vi "AlazarStackChannels1Pass.vi"(6 "AlazarCluster":T8, 7 "Digitizer Settings":T4 {"Trigger Settings"."Trig Slope" items=["Positive", "Negative"]; "Trigger Settings"."Level (mV)" format="%.2f"; "Trigger Settings"."Trig Coupling" items=["DC 1 MOhm", "AC 1 MOhm", "DC 50 Ohm", "AC 50 Ohm"]; "Trigger Settings"."Trig Source" items=["Chan 1", "External"]; "Rel Dig Delay" format="%.2f"; "DigTimeOut" format="%.2f"; "Avg Num" min=1; "Offset delay (us)" format="%.2f"; "Additional dig delay (us)" format="%.2f"; "Digitizer delay (us)" format="%.2f"}, 8 "error in":errorcluster, 10 "Extra Shift":u16, 11 "Ann Array Params":T1={"Synth Foc?"=FALSE, "Focal Zones"=41, "Switch T/R"=0, "Trans Geometry (mm)"={"Transducer"=0, "Geo Focus"=12.0, "a (radius)"=3.0, "# of rings"=5, "kerf space "=0.1, "Center Freq"=12.0}, "Sub Ap Excite?"=FALSE, "Full Array Scan?"=FALSE, "Xmt/Rcv"={"XMIT"=[TRUE, TRUE, TRUE, TRUE, TRUE], "RCV"=[TRUE, TRUE, TRUE, TRUE, TRUE]}, "PulseSpacing (us)"=0.0, "Xmit Ring"=0, "XMIT CHS"=0, "RCV CHS"=0, "GPU?"=FALSE, "Save TIFF?"=FALSE, "downfactor"=1, "RCV 1CH"=0} {"RCV 1CH" items=["All", "1", "2", "3", "4", "5"]; "Trans Geometry (mm)"."Transducer" items=["6D 12R 40 MHz"=0, "10D 31R 20 MHz"=1, "10D 23R 20 MHz"=2, "6D 23R 40 MHz"=3, "4.5D 10.7R 40 MHz"=4, "9D 23.5R 20 MHz"=5, "9D 25.8R 20MHz"=6, "Enter"=99]; "Switch T/R" min=1 max=5 step=1}) -> (0 "error out":errorcluster, 1 "Voltage Scale":dbl, 2 "Return Code":u32, 3 "DataInterleavedOut":i16[](array[numeric]), 4 "DeInterleaved":i16[](array[numeric]))   [LabVIEW 2022 SP3]
uses:
  -DigitizerRoutines/DigitizerSettings.ctl
  -DigitizerRoutines/Digitizer.ctl
  -DigitizerRoutines/DigConfig.ctl
  -DigitizerRoutines/DigitizerID.ctl
  C:/Windows/System32/ADQAPI_dotNet_helper.dll
  Annular Array/-AnnularRoutines/AnnularArray.ctl
  Annular Array/-AnnularRoutines/TransGeometry.ctl
  Annular Array/-AnnularRoutines/ArrayGeometry.ctl
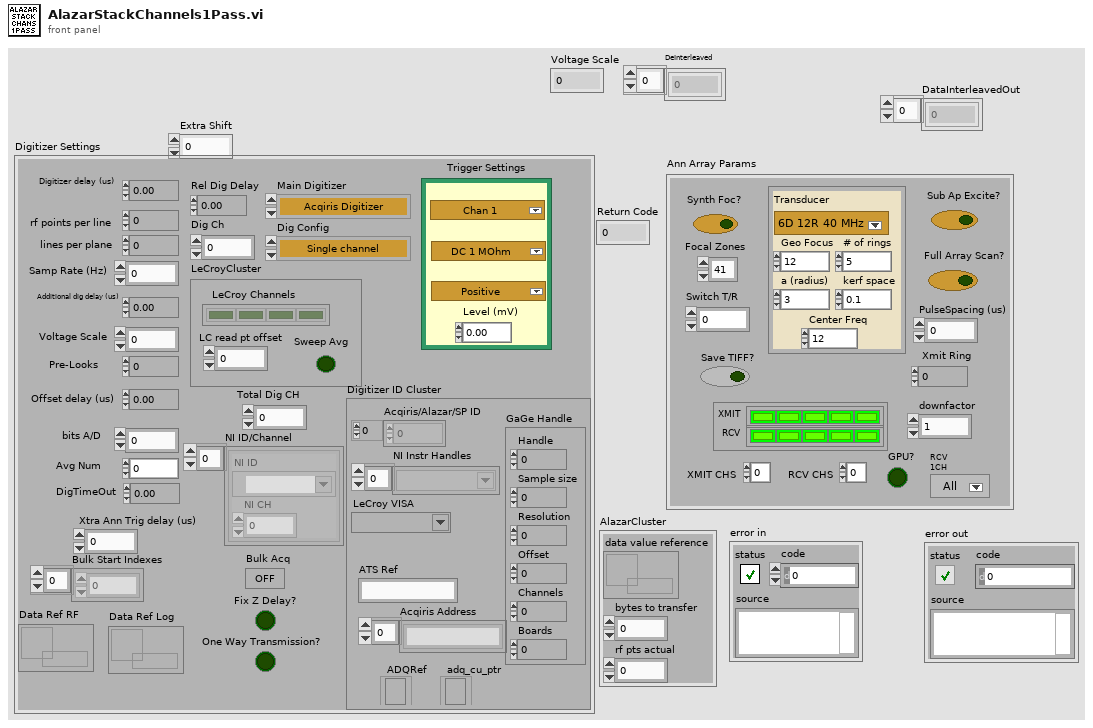
[diagram p1: front panel]
types:
  T1 = typedef "AnnularArray.ctl" = cluster{"Synth Foc?":bool, "Focal Zones":i16, "Switch T/R":i16, "Trans Geometry (mm)":T2, "Sub Ap Excite?":bool, "Full Array Scan?":bool, "Xmt/Rcv":cluster{"XMIT":bool[], "RCV":bool[]}, "PulseSpacing (us)":sgl, "Xmit Ring":i32, "XMIT CHS":u8, "RCV CHS":u8, "GPU?":bool, "Save TIFF?":bool, "downfactor":i32, "RCV 1CH":u16}
  T2 = typedef "TransGeometry.ctl" = cluster{"Transducer":T3, "Geo Focus":dbl, "a (radius)":dbl, "# of rings":i32, "kerf space ":dbl, "Center Freq":dbl}
  T3 = typedef "ArrayGeometry.ctl" = u16
  T4 = typedef "DigitizerSettings.ctl" = cluster{"Digitizer delay (us) ":dbl, "rf points per line":i32, "lines per plane":i32, "Samp Rate (Hz)":dbl, "Additional dig delay (us)":dbl, "Voltage Scale":dbl, "Pre-Looks":i32, "Offset delay (us)":dbl, "bits A/D":i8, "Avg Num":i32, "DigTimeOut":sgl, "Rel Dig Delay":sgl, "Dig Ch":i32, "LeCroyCluster":cluster{"LeCroy Channels":bool[], "LC read pt offset":dbl, "Sweep Avg":bool}, "Main Digitizer":T5, "Dig Config":T6, "Digitizer ID Cluster":T7, "Trigger Settings":cluster{"Trig Source":u16, "Trig Coupling":u16, "Trig Slope":u16, "Level (mV)":dbl}, "Bulk Acq":bool, "Bulk Start Indexes":i32[], "Data Ref RF":refnum<data-value>, "NI ID/Channel":cluster{"NI ID":refnum<k15>, "NI CH":i32}[], "Total Dig CH":i32, "Xtra Ann Trig delay (us)":dbl, "Fix Z Delay?":bool, "One Way Transmission?":bool, "Data Ref Log":refnum<data-value>}
  T5 = typedef "Digitizer.ctl" = enum16{"Acqiris Digitizer", "NI Digitizer", "LeCroy", "GaGe", "AlazarTech", "No Digitizer", "Teledyne"}
  T6 = typedef "DigConfig.ctl" = enum16{"Single channel", "2 Chans w/ 2 Acqiris", "2 Chans w/ 1 Acqiris", "5-CH Pulser New", "5-CH pulser w/ ann array", "5-pass style ann array", "Empty"}
  T7 = typedef "DigitizerID.ctl" = cluster{"Acqiris/Alazar/SP ID":u32[], "NI Instr Handles":refnum<k15>[], "LeCroy VISA":refnum<visa-resource-name>, "GaGe Handle":cluster{"Handle":u32, "Sample size":u32, "Resolution":i32, "Offset":i32, "Channels":u32, "Boards":u32}, "ATS Ref":string, "Acqiris Address":string[], "ADQRef":refnum<k24>, "adq_cu_ptr":refnum<k24>}
  T8 = cluster{"data value reference":refnum<data-value>, "bytes to transfer":u32, "rf pts actual":u32}
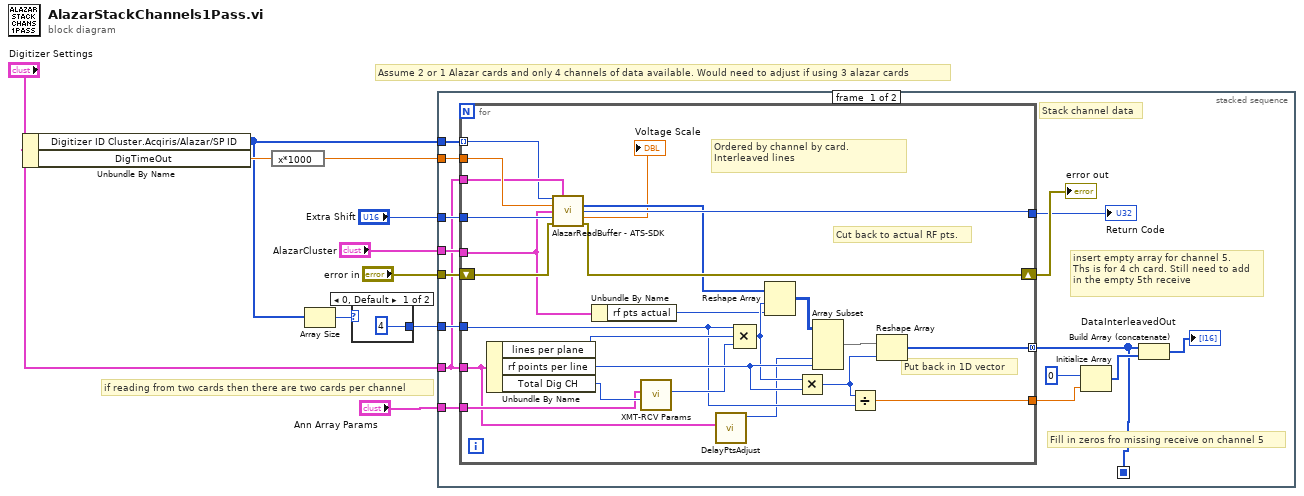
[diagram p0: block diagram]
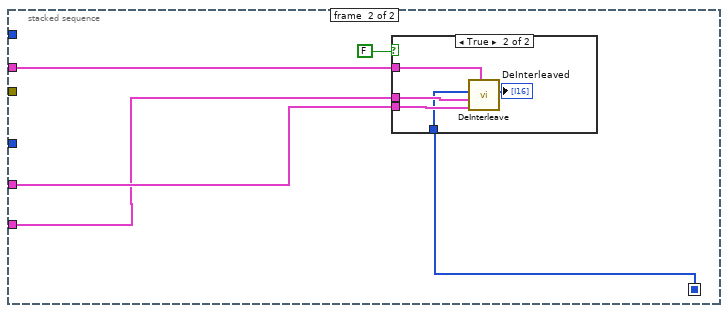
[diagram p2: hidden frame]
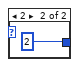
[diagram p4: hidden frame]
diagram:
  # "Assume 2 or 1 Alazar cards and only 4 channels of data available. Would need to adjust if using 3 alazar cards"
  # "if reading from two cards then there are two cards per channel"
  n1 = Unbundle By Name("Digitizer Settings") -> ("Digitizer ID Cluster.Acqiris/Alazar/SP ID"=w6:u32[], "DigTimeOut"=w7:sgl)
  n2 = expression code="x*1000"(w7) -> (w8:sgl)
  n3 = Array Size(array=w6) -> (size(s)=w2:i32)
  n4 = case shown="0, Default" w2 {
    tunnel: [4 ("y") 2 ("y")] -> w1
    frame 0, Default {
    }
    frame 2 {
    }
  }
  n5 = stacked-sequence {
    seq-local: [w13 _] -> [_ w56]
    tunnel: "error in" -> [w26 _]
    tunnel: "Extra Shift" -> [w25 _]
    tunnel: w8 -> [w24 _]
    tunnel: w6 -> [w23 _]
    tunnel: "AlazarCluster" -> [w21 w53]
    tunnel: "Digitizer Settings" -> [w14 w55]
    tunnel: "Ann Array Params" -> [w16 w54]
    tunnel: w1 -> [w15 _]
    frame #0 {
      # "insert empty array for channel 5.\nThs is for 4 ch card. Still need to add\nin the empty 5th receive"
      # "Fill in zeros fro missing receive on channel 5"
      # "Stack channel data"
      n6 = for {
        tunnel: w21 -> [w33]
        tunnel: w25 -> [w50]
        tunnel: w24 -> [w49]
        tunnel: w14 -> [w48]
        tunnel: w23 -> [w47] mode=indexing
        shift-right: [w52] -> w27
        shift-left: w26 -> [w51]
        tunnel: [w46] -> w22
        tunnel: w14 -> [w29]
        tunnel: w15 -> [w36]
        tunnel: [w35] -> w13 mode=concatenating
        tunnel: [w34] -> w20
        tunnel: w16 -> [w31]
        # "Ordered by channel by card. Interleaved lines"
        # "Put back in 1D vector"
        # "Cut back to actual RF pts."
        n7 = Unbundle By Name(w29) -> ("lines per plane"=w43:i32, "rf points per line"=w45:i32, "Total Dig CH"=w42:i32)
        n8 = call "AlazarReadBuffer - ATS-SDK.vi"("Handle"=w47, "Digitizer Settings"=w48, "time out (ms)"=w49, "AlazarCluster"=w33, "Extra Shift"=w50, "error in (no error)"=w51) -> ("Data Array"=w37:i16[], "Return Code"=w46:u32, "Voltage Scale"=→"Voltage Scale":dbl, "error out"=w52:errorcluster)  [unwired: 5 in, 1 out]
        n9 = Unbundle By Name(w33) -> ("rf pts actual"=w32:u32)
        n10 = call "XMT-RCV Params.vi"("Dig Channels"=w42, "Ann Array Params"=w31) -> ("# XMIT"=w44:i16)  [unwired: 4 in, 5 out]
        n11 = call "DelayPtsAdjust.vi"("Digitizer Settings"=w29) -> ("PostDelayCorrection"=w28:u32)  [unwired: 9 in, 1 out]
        n12 = Compound Arithmetic op=MULTIPLY(w36, w43, w44) -> (w38:i32)
        n13 = Reshape Array(w37, w38, w32) -> (w40:i16[][])
        n14 = Multiply(x=w38, y=w45) -> (x*y=w41:i32)
        n15 = Array Subset(array=w40, index (col)=w28, length (col)=w45) -> (w39:i16[][])  [unwired: 2 in]
        n16 = Divide(x=w41, y=w36) -> (x/y=w34:dbl)
        n17 = Reshape Array(w39, w41) -> (w35:i16[])
      }
      "error out" <- w27
      "Return Code" <- w22
      n18 = Initialize Array(i16 0, w20) -> (w19:i16[])
      n19 = Build Array (concatenate)(w13, w19) -> (→"DataInterleavedOut":i16[])
    }
    frame #1 {
      n20 = case shown="True" FALSE {
        tunnel: w56 -> [_ w59]
        tunnel: w55 -> [_ w62]
        tunnel: w54 -> [_ w61]
        tunnel: w53 -> [_ w60]
        frame False {
        }
        frame True {
          n21 = call "DeInterleave.vi"("AlazarCluster"=w60, "Digitizer Settings"=w62, "Ann Array Params"=w61, "Alazar Data"=w59) -> ("Sorted Array Out"=→"DeInterleaved":i16[])  [unwired: 7 in]
        }
      }
    }
  }
